vi "CAL-Apply Microphone Correction.vi"(0 "Correction curve":path, 5 "data":T1, 11 "error in (no error)":errorcluster) -> (6 "corrected data":T1, 15 "error out":errorcluster)   [LabVIEW 2020]
uses:
  Typedefs/CAL-Data.ctl
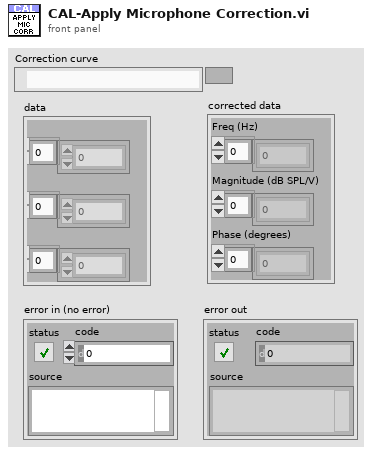
[diagram p1: front panel]
types:
  T1 = typedef "CAL-Data.ctl" = cluster{"Freq (Hz)":dbl[], "Magnitude (dB SPL/V)":dbl[], "Phase (degrees)":dbl[]}
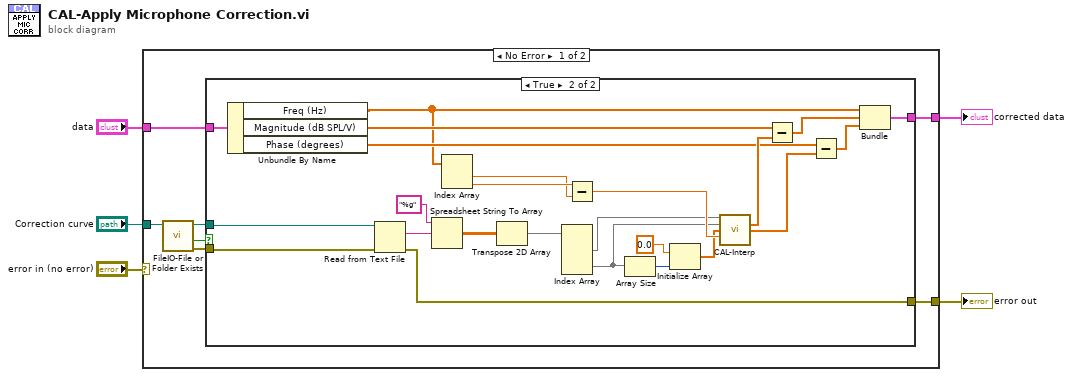
[diagram p0: block diagram]
diagram:
  n1 = case shown="No Error" "error in (no error)" {
    selector: "error in (no error)" -> [_ w40]
    tunnel: "Correction curve" -> [w12 _]
    tunnel: [w8 w40] -> w3
    tunnel: "data" -> [w7 w39]
    tunnel: [w6 w39] -> w1
    frame No Error {
      n2 = call "FileIO-File or Folder Exists.vi"("path"=w12) -> ("error out"=w9:errorcluster, "Exists?"=w10:bool, "dup path"=w11:path)  [unwired: 7 in, 1 out]
      n3 = case shown="True" w10 {
        tunnel: w11 -> [_ w33]
        tunnel: w9 -> [w14 w32]
        tunnel: [w14 w31] -> w8
        tunnel: w7 -> [w13 w21]
        tunnel: [w13 w15] -> w6
        frame False {
        }
        frame True {
          n4 = Unbundle By Name(w21) -> ("Freq (Hz)"=w18:dbl[], "Magnitude (dB SPL/V)"=w20:dbl[], "Phase (degrees)"=w19:dbl[])
          n5 = Read from Text File(file (use dialog)=w33, error in=w32) -> (text=w30:string, error out=w31:errorcluster)  [unwired: 2 in, 2 out]
          n6 = Spreadsheet String To Array(format string="%g", spreadsheet string=w30) -> (array=w29:dbl[][])  [unwired: 2 in]
          n7 = Index Array(array=w18) -> (element #1=w37:dbl, element #2=w38:dbl)  [unwired: 2 in]
          n8 = Transpose 2D Array(2D array=w29) -> (transposed array=w22:dbl[][])
          n9 = Index Array(array=w22) -> (element #1=w24:dbl[], element #2=w23:dbl[])  [unwired: 4 in]
          n10 = Subtract(x=w38, y=w37) -> (x-y=w36:dbl)
          n11 = Array Size(array=w23) -> (size(s)=w28:i32)
          n12 = Initialize Array(0.0, w28) -> (w26:dbl[])
          n13 = call "CAL-Interp.vi"("Frequency (Hz)"=w24, "Magnitude (dB)"=w23, "Phase (degrees)"=w26, "df (Hz)"=w36) -> ("Interp Magnitude (dB)"=w35:dbl[], "Interp Phase (degrees)"=w34:dbl[])  [unwired: 8 in, 2 out]
          n14 = Subtract(x=w20, y=w35) -> (x-y=w17:dbl[])
          n15 = Subtract(x=w19, y=w34) -> (x-y=w16:dbl[])
          n16 = Bundle("Freq (Hz)"=w18, w17, w16) -> (w15:cluster{"Freq (Hz)":dbl[], dbl[], dbl[]})  [unwired: 1 in]
        }
      }
    }
    frame Error {
    }
  }
  "error out" <- w3
  "corrected data" <- w1
